vi "Add to Database Button Constructor.vi"(8 "error in (no error)":errorcluster, 9 "Ctl Refnum":refnum<vi>, 10 "Self Enqueuer":refnum<class "Message Enqueuer.lvclass">, 11 "Add Form to Database Button in":refnum<class "Add Form to Database Button.lvclass">) -> (0 "error out":errorcluster, 3 "Add Form to Database Button out":refnum<class "Add Form to Database Button.lvclass">)   [LabVIEW 2020, in "Panel Form Controller.lvlib" / "Add Form to Database Button.lvclass"]
uses:
  Add Form to Database Button.lvclass
  C:/Users/User/Desktop/Raman Program/Database OOP/source/Database OOP/Button Libraries/Button/Button Class/Button.lvclass
  <vilib>/ActorFramework/Message Enqueuer/Message Enqueuer.lvclass
  Database OOP/Button Libraries/Button/Button Class/Button.lvclass/Button.ctl
  Add Form to Database Button.lvclass/Add Form to Database Button.ctl
  Database OOP/Button Libraries/Button/Button Class/Button.lvclass
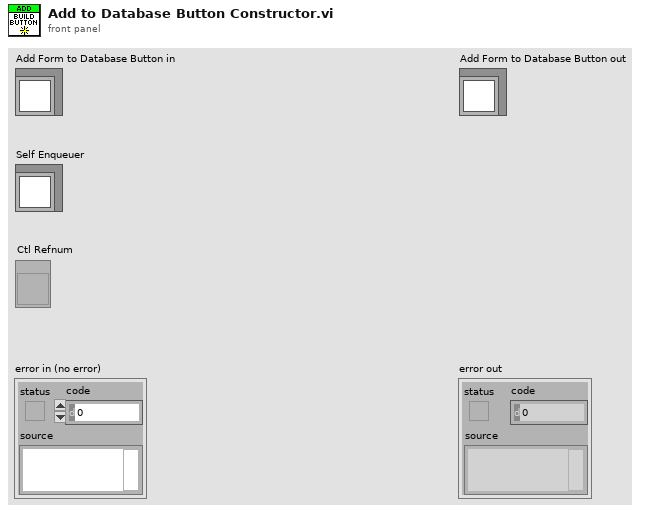
[diagram p1: front panel]
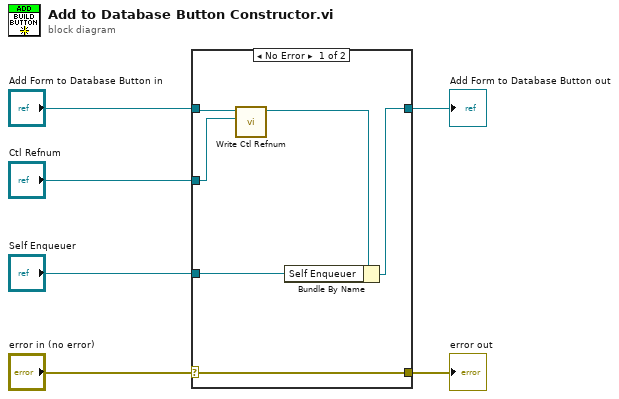
[diagram p0: block diagram]
diagram:
  n1 = case shown="No Error" "error in (no error)" {
    selector: "error in (no error)" -> [w12 w14]
    tunnel: [w12 w14] -> w5
    tunnel: [w9 w13] -> w3
    tunnel: "Add Form to Database Button in" -> [w11 w13]
    tunnel: "Self Enqueuer" -> [w8 _]
    tunnel: "Ctl Refnum" -> [w7 _]
    frame No Error {
      n2 = call "Write Ctl Refnum.vi"("Ctl Refnum"=w7, "Button in"=w11) -> ("Button out"=w10:refnum<class "Add Form to Database Button.lvclass">)  [unwired: 8 in, 1 out]
      n3 = Bundle By Name(cluster=w10, "Self Enqueuer"=w8) -> (w9:refnum<class "Add Form to Database Button.lvclass">)
    }
    frame Error {
    }
  }
  "error out" <- w5
  "Add Form to Database Button out" <- w3
